vi "auto_constSpeedNoLoad.vi"(10 "speed":dbl, 11 "Speed":i32) -> (2 "Pass":bool, 3 "Set speed":i32, 5 "torque":sgl)   [LabVIEW 2019]
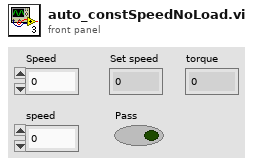
[diagram p1: front panel]
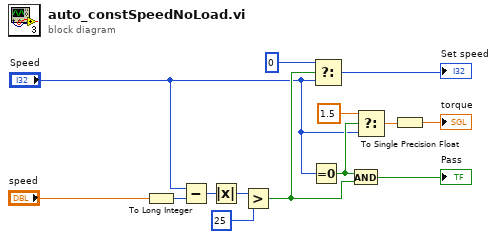
[diagram p0: block diagram]
diagram:
  n1 = To Long Integer(number="speed") -> (32bit integer=w11:i32)
  n2 = Subtract(x="Speed", y=w11) -> (x-y=w12:i32)
  n3 = Absolute Value(x=w12) -> (abs(x)=w14:i32)
  n4 = Greater?(x=w14, y=25) -> (0:w7:bool)
  n5 = Equal To 0?(x="Speed") -> (x = 0?=w5:bool)
  n6 = Select(t=0, s=w7, f="Speed") -> (s? t:f=→"Set speed":i32)
  n7 = And(x=w5, y=w7) -> (x .and. y?=→"Pass":bool)
  n8 = Select(t=1.5, s=w5, f="Speed") -> (s? t:f=w2:dbl)
  n9 = To Single Precision Float(number=w2) -> (single precision float=→"torque":sgl)
